vi "Get king square by color.vi"(8 "error in (no error)":errorcluster, 10 "Color":T4, 11 "Board in":refnum<class "Board.lvclass">) -> (0 "error out":errorcluster, 1 "found?":bool, 2 "Square":T1={"File"=enum."d", "Rank"=enum."4"}, 3 "Board out":refnum<class "Board.lvclass">)   [LabVIEW 2016, in "Chesslib.lvlib" / "Board.lvclass"]
uses:
  Board.lvclass
  typedef/Color.ctl
  typedef/Square.ctl
  typedef/File.ctl
  typedef/Rank.ctl
  Board.lvclass/Board.ctl
  typedef/Piece type.ctl
  Pieces/Piece/Piece.lvclass/Piece.ctl
  <vilib>/Utility/error.llb/Error Cluster From Error Code.vi
  <vilib>/ErrorRing/Error Ring.xnode
  Pieces/Piece/Piece.lvclass
  Chesslib.lvlib
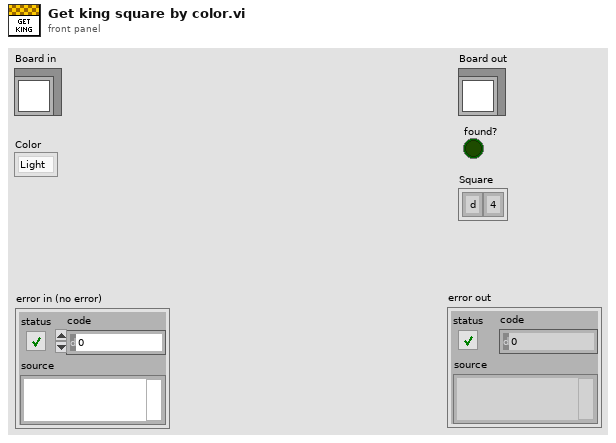
[diagram p1: front panel]
types:
  T1 = typedef "Chesslib.lvlib/Square.ctl" = cluster{"File":T2, "Rank":T3}
  T2 = typedef "Chesslib.lvlib/File.ctl" = enum8{"a", "b", "c", "d", "e", "f", "g", "h"}
  T3 = typedef "Chesslib.lvlib/Rank.ctl" = enum8{"1", "2", "3", "4", "5", "6", "7", "8"}
  T4 = typedef "Chesslib.lvlib/Color.ctl" = enum16{"Light", "Dark"}
  T5 = typedef "Chesslib.lvlib/Piece type.ctl" = enum16{"Pawn", "Bishop", "Knight", "Rook", "Queen", "King"}
  T6 = typedef "Chesslib.lvlib/Board.lvclass/Square content.ctl" = cluster{"Occupied":bool, "Piece":refnum<class "Piece.lvclass">}
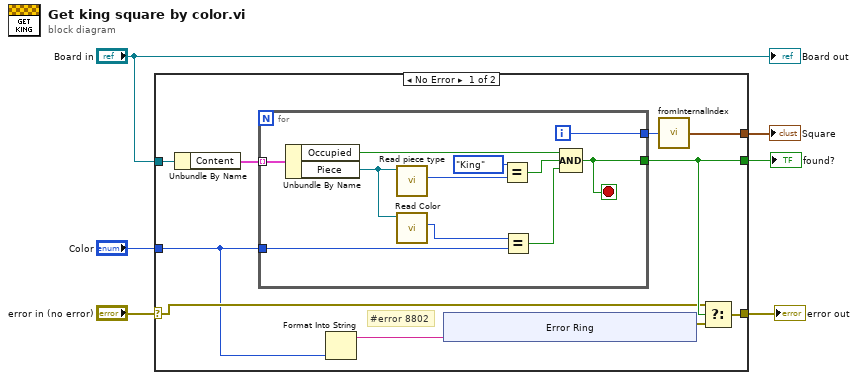
[diagram p0: block diagram]
diagram:
  n1 = case shown="No Error" "error in (no error)" {
    selector: "error in (no error)" -> [w10 w35]
    tunnel: "Color" -> [w9 _]
    tunnel: "Board in" -> [w15 _]
    tunnel: [w11 _] -> w4
    tunnel: [w13 _] -> w3
    tunnel: [w12 w35] -> w2
    frame No Error {
      # "#error 8802"
      n2 = Unbundle By Name(w15) -> ("Content"=w16:T6[])
      n3 = for {
        tunnel: w16 -> [w27] mode=indexing
        tunnel: w9 -> [w25]
        tunnel: [w20] -> w14
        tunnel: [w21] -> w11
        i -> [w20]
        stop <- w21 stop-if-true
        n4 = Unbundle By Name(w27) -> ("Occupied"=w26:bool, "Piece"=w18:refnum<class "Piece.lvclass">)
        n5 = call-dynamic "Read piece type.vi"("Piece in"=w18) -> ("Piece type"=w19:T5)  [unwired: 10 in]
        n6 = call "Read Color.vi"("Piece in"=w18) -> ("Color"=w17:T4)  [unwired: 10 in]
        n7 = Equal?(x=Piece_type."King", y=w19) -> (x = y?=w22:bool)
        n8 = Equal?(x=w17, y=w25) -> (x = y?=w24:bool)
        n9 = Compound Arithmetic op=AND(w26, w22, w24) -> (w21:bool)
      }
      n10 = Format Into String(w9) -> (resulting string=w8:string)  [unwired: 3 in, 1 out]
      n11 = xnode "Error Ring"("parameter 0"=w8) -> ("error out"=w7:errorcluster)
      n12 = call "fromInternalIndex.vi"("Internal index"=w14) -> ("Square"=w13:T1)
      n13 = Select(t=w10, s=w11, f=w7) -> (s? t:f=w12:errorcluster)
    }
    frame Error {
    }
  }
  "Square" <- w3
  "found?" <- w4
  "error out" <- w2
  "Board out" <- "Board in"
